vi "GSTOP GET.vi"(1 "index(-1 for All)":i32=-1, 7 "error in (no error)":errorcluster) -> (6 "stop":bool, 8 "error out":errorcluster)   [LabVIEW 2017, in "GSTOP.lvlib"]
doc: "Reads a stop flag by index; Index=-1 means read the global stop flag.\n------\n读取指定索引的停止位；Index=-1 表示读取全局停止位。"
uses:
  GSTOP.lvlib
  _def_oper.ctl
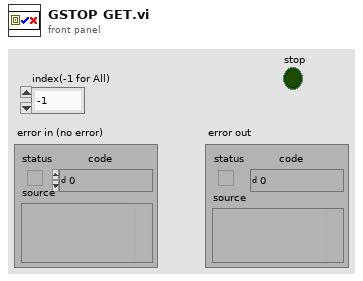
[diagram p1: front panel]
types:
  T1 = typedef "GSTOP.lvlib/_def_oper.ctl" = enum16{"init", "reset", "get", "set"}
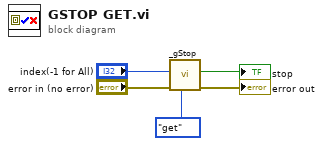
[diagram p0: block diagram]
diagram:
  n1 = call "_gStop.vi"("op"=_def_oper."get", "error in (no error)"="error in (no error)", "index(-1 for All)"="index(-1 for All)") -> ("error out"=→"error out":errorcluster, "stop"=→"stop":bool)  [unwired: 7 in]
